vi "ECSE421_lab1.vi"() -> ()   [LabVIEW 2017]
panel:
  in  "stop":bool
  in  "Grab soda (reset)":bool
  out "Change deposited":string
  out "Change returned":string
  out "Soda dispensed":bool
  in  "Quarter":bool
  in  "Dime":bool
  in  "Nickel":bool
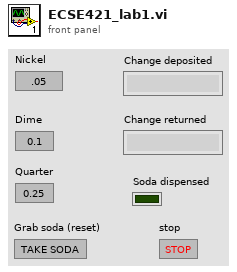
[diagram p1: front panel]
types:
  T1 = enum16{"0", "5", "10", "15", "20", "25", "30", "35", "40", "45"}
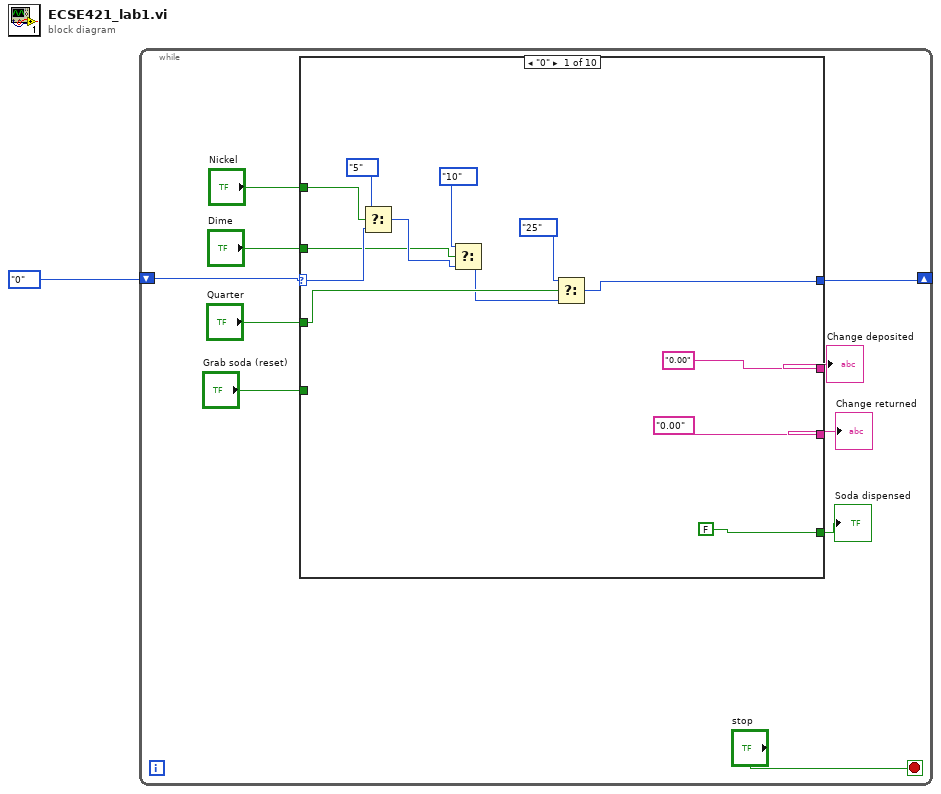
[diagram p0: block diagram]
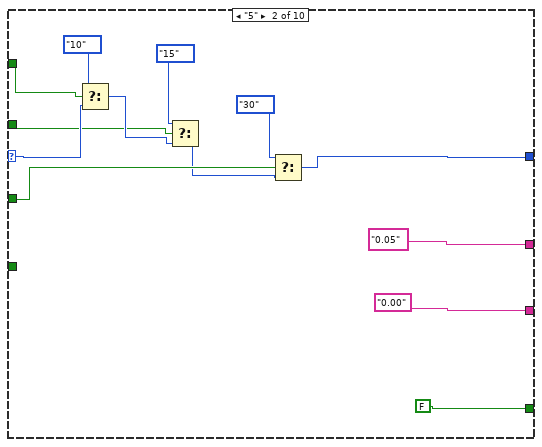
[diagram p2: hidden frame]
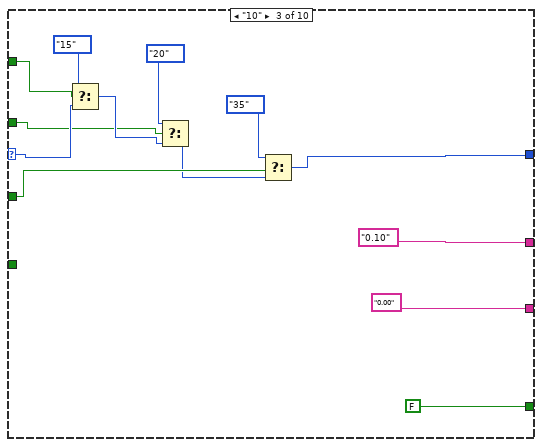
[diagram p3: hidden frame]
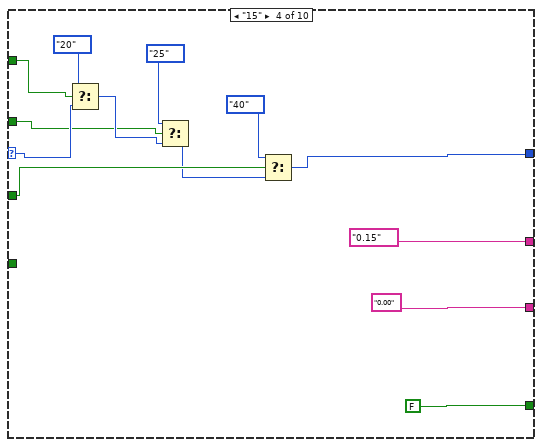
[diagram p4: hidden frame]
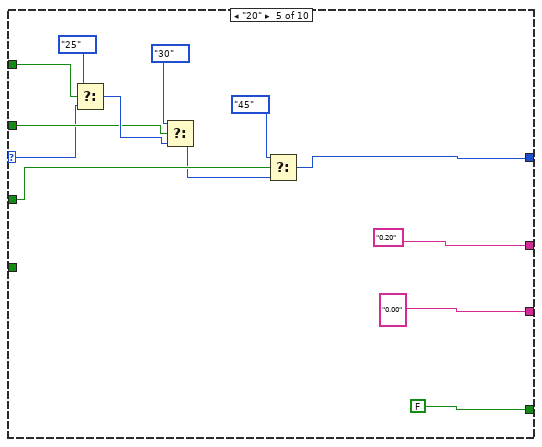
[diagram p5: hidden frame]
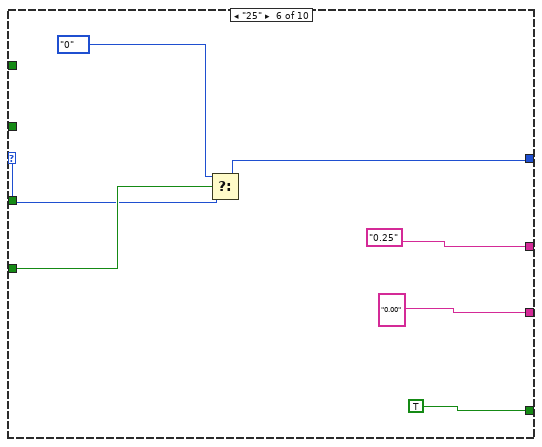
[diagram p6: hidden frame]
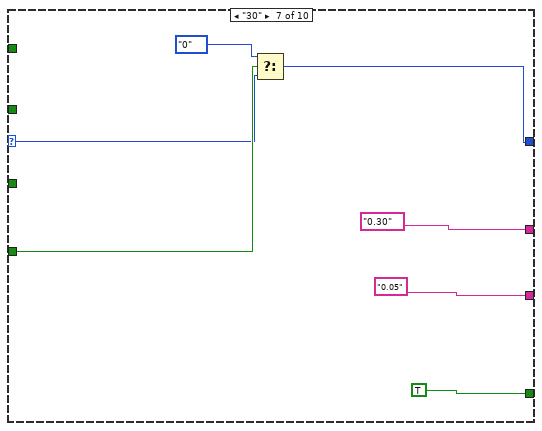
[diagram p7: hidden frame]
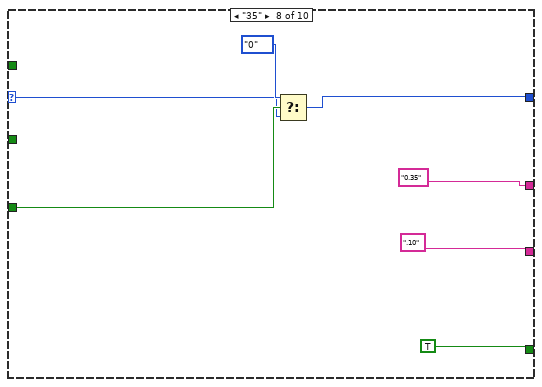
[diagram p8: hidden frame]
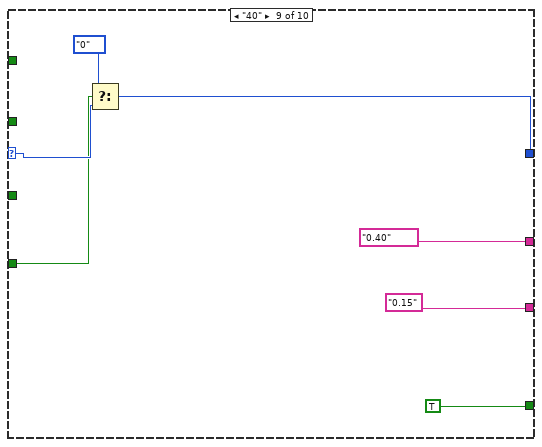
[diagram p9: hidden frame]
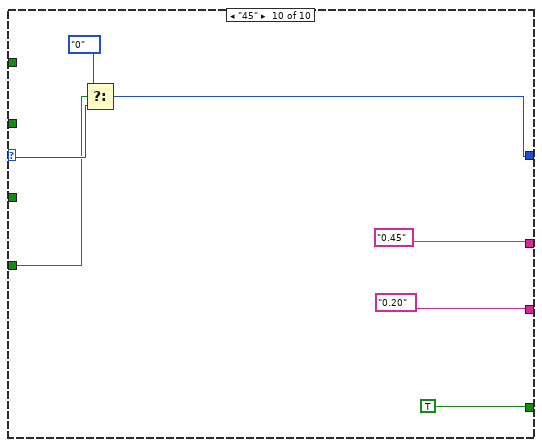
[diagram p10: hidden frame]
diagram:
  n1 = while {
    shift-right: [w3] -> _
    shift-left: T1."0" -> [w2]
    stop <- "stop" stop-if-true
    n2 = case shown="\"0\"" w2 {
      selector: w2 -> [w24 w33 w42 w59 w71 w77 w86 w91 w103 w110]
      tunnel: "Nickel" -> [w23 w31 w40 w57 w73 _ _ _ _ _]
      tunnel: "Dime" -> [w21 w32 w41 w58 w72 _ _ _ _ _]
      tunnel: "Quarter" -> [w20 w34 w43 w60 w70 _ _ _ _ _]
      tunnel: "Grab soda (reset)" -> [_ _ _ _ _ w79 w87 w93 w99 w106]
      tunnel: [w19 w30 w47 w55 w69 w78 w84 w97 w98 w105] -> w3
      tunnel: ["0.00" "0.05" "0.10" "0.15" "0.20" "0.25" "0.30" "0.35" "0.40" "0.45"] -> w7
      tunnel: ["0.00" "0.00" "0.00" "0.00" "0.00" "0.00" "0.05" ".10" "0.15" "0.20"] -> w6
      tunnel: [FALSE FALSE FALSE FALSE FALSE TRUE TRUE TRUE TRUE TRUE] -> w5
      frame "0" {
        n3 = Select(t=T1."5", s=w23, f=w24) -> (s? t:f=w22:T1)
        n4 = Select(t=T1."10", s=w21, f=w22) -> (s? t:f=w13:T1)
        n5 = Select(t=T1."25", s=w20, f=w13) -> (s? t:f=w19:T1)
      }
      frame "5" {
        n6 = Select(t=T1."10", s=w31, f=w33) -> (s? t:f=w35:T1)
        n7 = Select(t=T1."15", s=w32, f=w35) -> (s? t:f=w26:T1)
        n8 = Select(t=T1."30", s=w34, f=w26) -> (s? t:f=w30:T1)
      }
      frame "10" {
        n9 = Select(t=T1."15", s=w40, f=w42) -> (s? t:f=w48:T1)
        n10 = Select(t=T1."20", s=w41, f=w48) -> (s? t:f=w39:T1)
        n11 = Select(t=T1."35", s=w43, f=w39) -> (s? t:f=w47:T1)
      }
      frame "15" {
        n12 = Select(t=T1."20", s=w57, f=w59) -> (s? t:f=w61:T1)
        n13 = Select(t=T1."25", s=w58, f=w61) -> (s? t:f=w51:T1)
        n14 = Select(t=T1."40", s=w60, f=w51) -> (s? t:f=w55:T1)
      }
      frame "20" {
        n15 = Select(t=T1."25", s=w73, f=w71) -> (s? t:f=w74:T1)
        n16 = Select(t=T1."30", s=w72, f=w74) -> (s? t:f=w65:T1)
        n17 = Select(t=T1."45", s=w70, f=w65) -> (s? t:f=w69:T1)
      }
      frame "25" {
        n18 = Select(t=T1."0", s=w79, f=w77) -> (s? t:f=w78:T1)
      }
      frame "30" {
        n19 = Select(t=T1."0", s=w87, f=w86) -> (s? t:f=w84:T1)
      }
      frame "35" {
        n20 = Select(t=T1."0", s=w93, f=w91) -> (s? t:f=w97:T1)
      }
      frame "40" {
        n21 = Select(t=T1."0", s=w99, f=w103) -> (s? t:f=w98:T1)
      }
      frame "45" {
        n22 = Select(t=T1."0", s=w106, f=w110) -> (s? t:f=w105:T1)
      }
    }
    "Change deposited" <- w7
    "Change returned" <- w6
    "Soda dispensed" <- w5
  }
